vi "Method_Const.vi"(4 "Value":cdb, 5 "Value A":refnum<class "Abs_Complex Double Float.lvclass">) -> (1 "Result":refnum<class "Abs_Boolean.lvclass">)   [LabVIEW 2021, in "Not Equal_CPLX_DBL.lvclass"]
uses:
  Not Equal_CPLX_DBL.lvclass
  Abs_Types/Complex Double Float/Abs_Complex Double Float.lvclass
  C:/Program Files (x86)/National Instruments/LabVIEW 2021/vi.lib/TSA/Abstract Data Classes/Abs_Types/Numeric/Abs_Numeric.lvclass
  Abs_Types/Boolean/Abs_Boolean.lvclass
  C:/TSA/LV_Abstract/Source/Functions/Support/Compare/Two Term/CPLX_DBL/AbsComp_Two Term_CPLX_DBL.lvclass
  C:/Program Files (x86)/National Instruments/LabVIEW 2021/vi.lib/TSA/Abstract Data Classes/Abs_Types/Boolean/Abs_Boolean.lvclass
  Support/Compare/Two Term/CPLX_DBL/AbsComp_Two Term_CPLX_DBL.lvclass/AbsComp_Two Term_CPLX_DBL.ctl
  Support/Compare/Two Term/CPLX_DBL/Properties/Write Numeric A.vi
  Support/Compare/Two Term/CPLX_DBL/Properties/Write Numeric B.vi
  Constants/Support/CPLX_DBL/Const_CPLX_DBL.lvclass
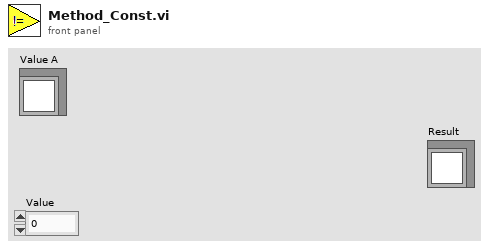
[diagram p1: front panel]
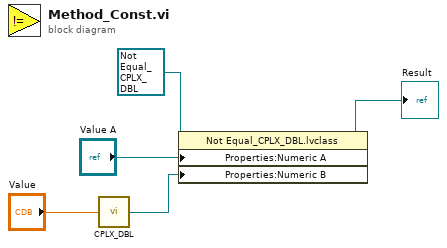
[diagram p0: block diagram]
diagram:
  n1 = call "CPLX_DBL.vi"("Value"="Value") -> ("Constant"=w2:refnum<class "Abs_Complex Double Float.lvclass">)  [unwired: 4 in]
  n2 = property class="Not Equal_CPLX_DBL.lvclass"(reference=refnum<class "Not Equal_CPLX_DBL.lvclass"> refnum ("Greater 0_U64.lvclass"), "Properties:Numeric A"="Value A", "Properties:Numeric B"=w2) -> (reference out=→"Result":refnum<class "Not Equal_CPLX_DBL.lvclass">)  [unwired: 1 in, 1 out]
